vi "AlazarGetStatus.vi"(0 "Handle":u64, 5 "error in (no error)":errorcluster) -> (14 "Handle":u64, 15 "Trig. Timeout":bool, 16 "Chan. A out of range":bool, 17 "Chan. B out of range":bool, 18 "PLL Locked":bool, 19 "error out":errorcluster)   [LabVIEW 2009]
doc: "Return a bitmask with board status information."
uses:
  ATSApi.dll
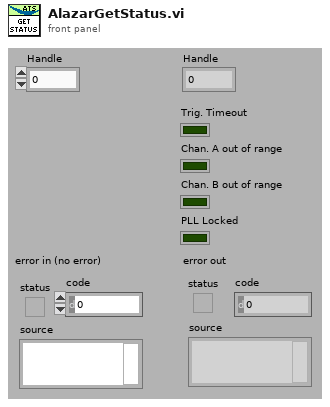
[diagram p1: front panel]
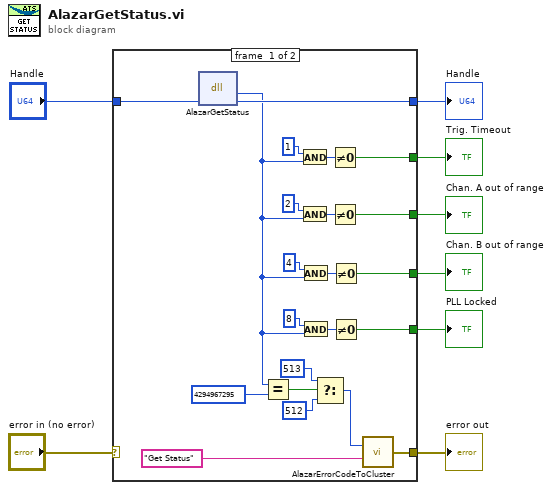
[diagram p0: block diagram]
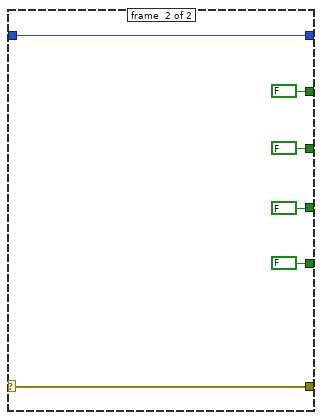
[diagram p2: hidden frame]
diagram:
  n1 = case shown="No Error" "error in (no error)" {
    selector: "error in (no error)" -> [_ w36]
    tunnel: [w28 w36] -> w7
    tunnel: "Handle" -> [w30 w35]
    tunnel: [w27 w35] -> w5
    tunnel: [w12 FALSE] -> w4
    tunnel: [w11 FALSE] -> w3
    tunnel: [w10 FALSE] -> w2
    tunnel: [w9 FALSE] -> w1
    frame #0 {
      n2 = dll-call lib="ATSApi.dll" fn="AlazarGetStatus"("handle"=w30) -> ("return type"=w13:u32, "handle"=w27:u64)  [unwired: 3 in, 2 out]
      n3 = Equal?(x=w13, y=u32 4294967295) -> (x = y?=w25:bool)
      n4 = And(x=u32 1, y=w13) -> (x .and. y?=w20:u32)
      n5 = And(x=u32 2, y=w13) -> (x .and. y?=w18:u32)
      n6 = And(x=u32 4, y=w13) -> (x .and. y?=w16:u32)
      n7 = And(x=u32 8, y=w13) -> (x .and. y?=w14:u32)
      n8 = Select(t=u32 513, s=w25, f=u32 512) -> (s? t:f=w22:u32)
      n9 = Not Equal To 0?(x=w20) -> (x != 0?=w12:bool)
      n10 = Not Equal To 0?(x=w18) -> (x != 0?=w11:bool)
      n11 = Not Equal To 0?(x=w16) -> (x != 0?=w10:bool)
      n12 = Not Equal To 0?(x=w14) -> (x != 0?=w9:bool)
      n13 = call "AlazarErrorCodeToCluster.vi"("Message"="Get Status", "Error Code"=w22) -> ("error out"=w28:errorcluster)
    }
    frame #1 {
    }
  }
  "Handle" <- w5
  "error out" <- w7
  "Chan. B out of range" <- w2
  "PLL Locked" <- w1
  "Chan. A out of range" <- w3
  "Trig. Timeout" <- w4
